vi "0620A.vi"() -> ()   [LabVIEW 2013]
panel:
  out "Data":u8[](array[numeric]) format="%x"
  out "Result":string
  in  "CMD":u8=1
  in  "Length":u8=7
  in  "ID":u8=1
  in  "Time":u16=1000 max=30000 step=1
  in  "Pos":dbl min=0.0 max=240.0 step=0.24
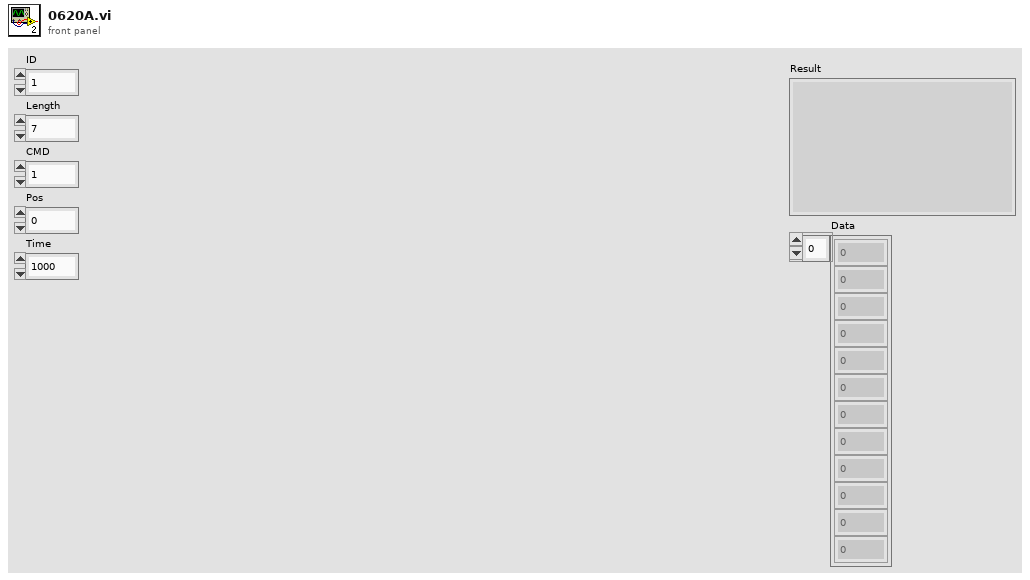
[diagram p1: front panel]
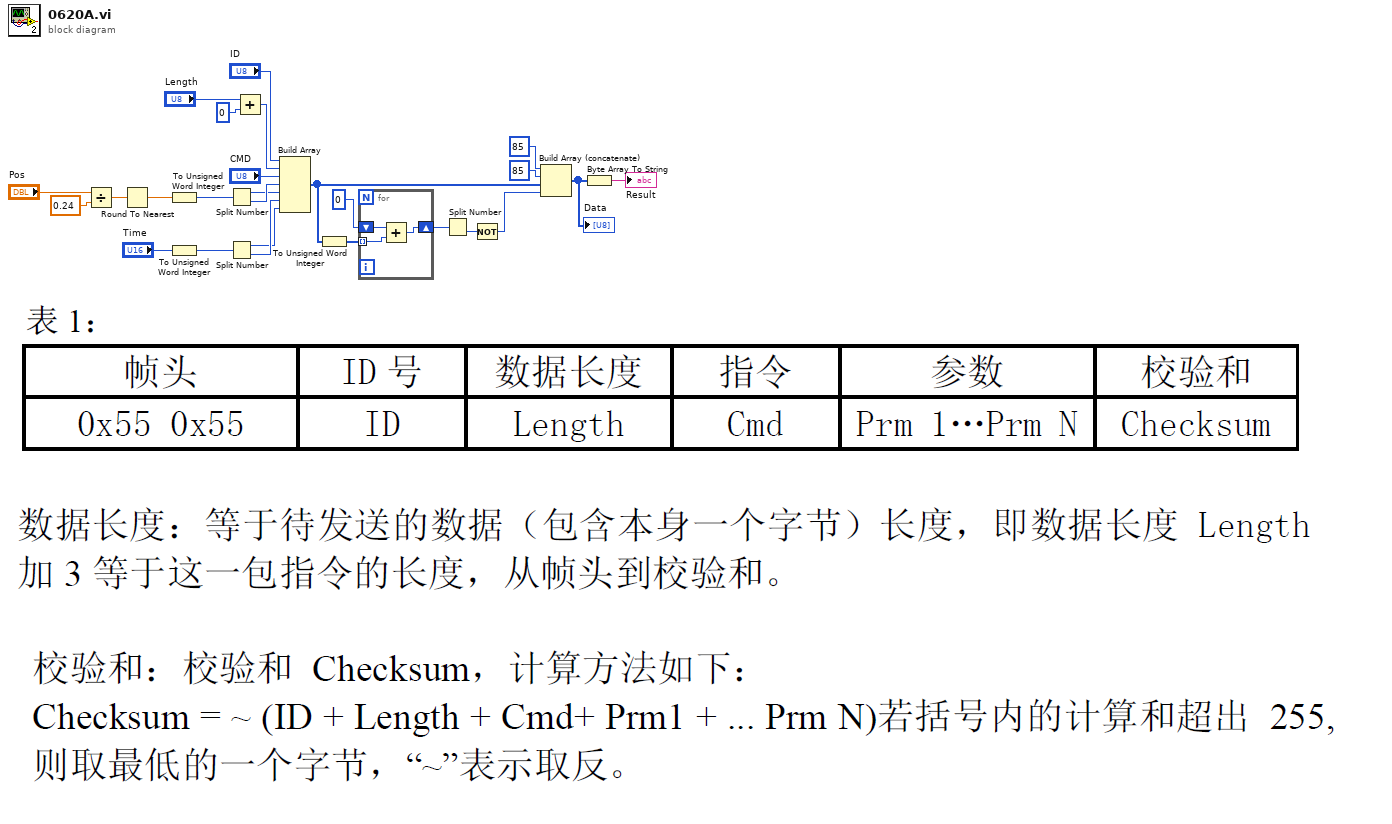
[diagram p0: block diagram]
diagram:
  n1 = Divide(x="Pos", y=0.24) -> (x/y=w26:dbl)
  n2 = Round To Nearest(number=w26) -> (nearest integer value=w25:dbl)
  n3 = To Unsigned Word Integer(number=w25) -> (unsigned 16bit integer=w24:u16)
  n4 = To Unsigned Word Integer(number="Time") -> (unsigned 16bit integer=w21:u16)
  n5 = Split Number(x=w24) -> (hi(x)=w16:u8, lo(x)=w17:u8)
  n6 = Split Number(x=w21) -> (hi(x)=w14:u8, lo(x)=w15:u8)
  n7 = Add(x="Length", y=u8 0) -> (x+y=w5:u8)
  n8 = Build Array("ID", w5, "CMD", w17, w16, w15, w14) -> (w10:u8[])
  n9 = To Unsigned Word Integer(number=w10) -> (unsigned 16bit integer=w12:u16[])
  n10 = for {
    shift-right: [w27] -> w3
    shift-left: u16 0 -> [w29]
    tunnel: w12 -> [w28] mode=indexing
    n11 = Add(x=w29, y=w28) -> (x+y=w27:u16)
  }
  n12 = Split Number(x=w3) -> (lo(x)=w2:u8)  [unwired: 1 out]
  n13 = Not(x=w2) -> (.not. x?=w1:u8)
  n14 = Build Array (concatenate)(u8 85, u8 85, w10, w1) -> (w9:u8[])
  "Data" <- w9
  n15 = Byte Array To String(unsigned byte array=w9) -> (string=→"Result":string)
